vi "Execute.vi"(8 "error in (no error)":errorcluster, 9 "Consumer Queues in":T1, 10 "UI Process Command in":refnum<class "Update UI Status.lvclass">, 11 "UI Process Data in":T2) -> (0 "error out":errorcluster, 1 "Consumer Queues out":T1, 2 "Stop?":bool, 3 "UI Process Data out":T2)   [LabVIEW 2019, in "User Interface Process.lvlib" / "Update UI Status.lvclass"]
uses:
  Update UI Status.lvclass
  C:/Users/wg/Documents/LV_Projects/TestStand/App/UI Process/Generic UI Command/Generic UI Process Command.lvclass
  UI Process Data.ctl
  TS Framework/ExeLogging/UI Logger/UI Logger.lvclass
  UI State.ctl
  TS Framework/Consumer Queues.ctl
  Generic UI Command/Generic UI Process Command.lvclass
  DAC Process/Generic DAC Command/Generic DAC Process Command.lvclass
  Trig Process/Generic Trig Command/Generic Trig Process Command.lvclass
  Update UI Status.lvclass/Update UI Status.ctl
  User Interface Process.lvlib
  TS Framework/TS Framework.lvlib
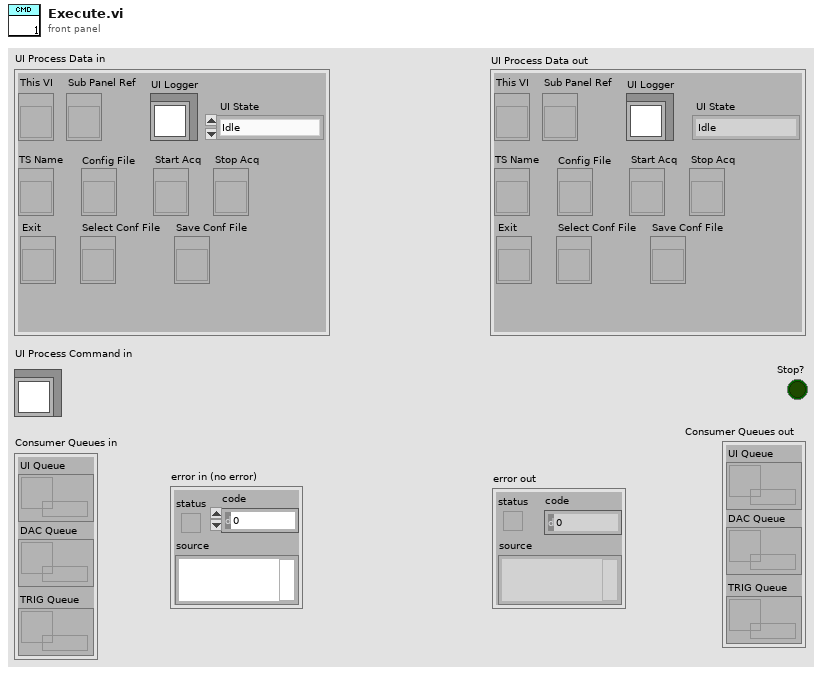
[diagram p1: front panel]
types:
  T1 = typedef "TS Framework.lvlib/Consumer Queues.ctl" = cluster{"UI Queue":refnum<queue>, "DAC Queue":refnum<queue>, "TRIG Queue":refnum<queue>}
  T2 = typedef "User Interface Process.lvlib/UI Process Data.ctl" = cluster{"This VI":refnum<vi>, "Sub Panel Ref":refnum<vi>, "UI Logger":refnum<class "UI Logger.lvclass">, "TS Name":refnum<vi>, "Config File":refnum<vi>, "Start Acq":refnum<vi>, "Stop Acq":refnum<vi>, "Exit":refnum<vi>, "Select Conf File":refnum<vi>, "Save Conf File":refnum<vi>, "UI State":T3}
  T3 = typedef "User Interface Process.lvlib/UI State.ctl" = enum16{"Idle", "Acquiring"}
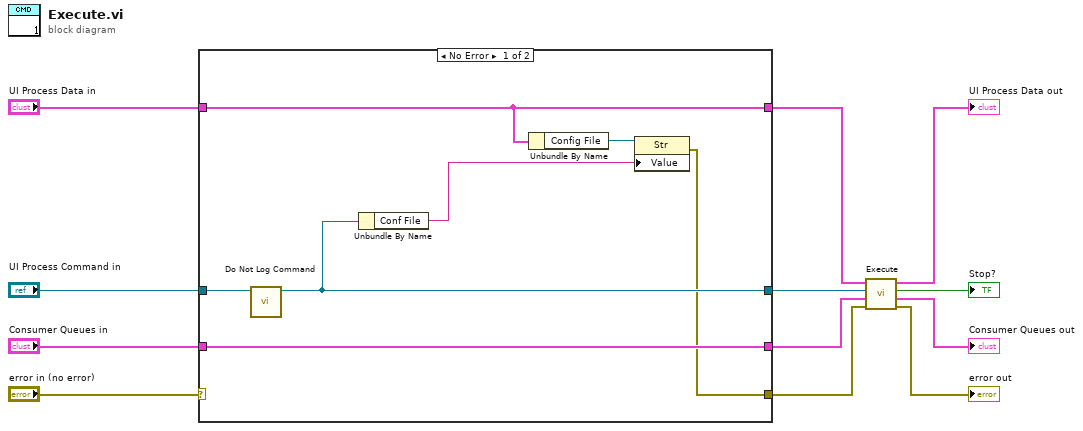
[diagram p0: block diagram]
diagram:
  n1 = case shown="No Error" "error in (no error)" {
    selector: "error in (no error)" -> [_ w20]
    tunnel: "UI Process Command in" -> [w19 w23]
    tunnel: "UI Process Data in" -> [w16 w22]
    tunnel: [w17 w23] -> w6
    tunnel: [w16 w22] -> w4
    tunnel: "Consumer Queues in" -> [w15 w21]
    tunnel: [w15 w21] -> w2
    tunnel: [w14 w20] -> w1
    frame No Error {
      n2 = call "Do Not Log Command.vi"("UI Process Command in"=w19) -> ("UI Process Command out"=w17:refnum<class "Update UI Status.lvclass">)  [unwired: 10 in]
      n3 = Unbundle By Name(w17) -> ("Conf File"=w13:string)
      n4 = Unbundle By Name(w16) -> ("Config File"=w18:refnum<vi>)
      n5 = property class="Str"(reference=w18, "Value"=w13) -> (error out=w14:errorcluster)  [unwired: 1 in, 1 out]
    }
    frame Error {
    }
  }
  n6 = call-parent "Execute.vi"("error in (no error)"=w1, "Consumer Queues in"=w2, "UI Process Command in"=w6, "UI Process Data in"=w4) -> ("error out"=→"error out":errorcluster, "Consumer Queues out"=→"Consumer Queues out":T1, "Stop?"=→"Stop?":bool, "UI Process Data out"=→"UI Process Data out":T2)  [unwired: 4 in]
